vi "LSCI332 SetPID.vi"(0 "VISA Rsrc":refnum<visa-resource-name>="GPIB0::12::INSTR", 5 "Boucle(1)":u32(ring) caption="Boucle" items=["Boucle 1", "Boucle 2"], 9 "Paramètres PID":cluster{"P":dbl, "I":dbl, "D":u32}={"P"=1000.0, "I"=0.0, "D"=0} {"D" max=200 step=1; "I" min=0.1 max=1000.0 step=0.1 format="%#.1f"; "P" min=0.1 max=1000.0 step=0.1 format="%#.1f"}, 11 "error in (no error)":errorcluster) -> (15 "error out":errorcluster)   [LabVIEW 2019]
doc: "Ce VI écrit les paramètres de la zone de contrôle spécifiée dans le contrôlleur"
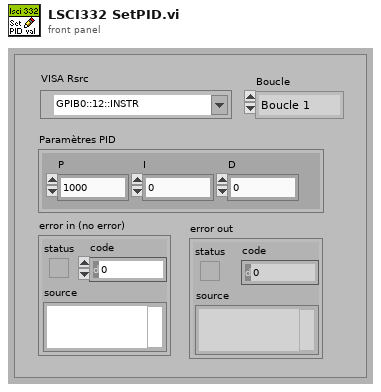
[diagram p1: front panel]
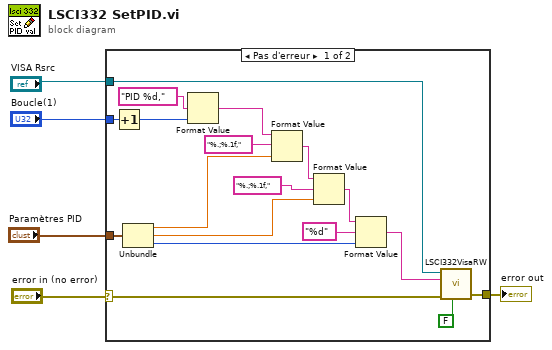
[diagram p0: block diagram]
diagram:
  n1 = case shown="Pas d'erreur" "error in (no error)" {
    selector: "error in (no error)" -> [w11 w24]
    tunnel: "VISA Rsrc" -> [w23 _]
    tunnel: "Boucle(1)" -> [w21 _]
    tunnel: [w22 w24] -> w3
    tunnel: "Paramètres PID" -> [w15 _]
    frame No Error {
      n2 = Increment(x=w21) -> (x+1=w16:u32)
      n3 = Unbundle(w15) -> ("P"=w14:dbl, "I"=w13:dbl, "D"=w12:u32)
      n4 = Format Value(format string="PID %d,", value (0)=w16) -> (output string=w9:string)  [unwired: 1 in]
      n5 = Format Value(string ("")=w9, format string="%.;%.1f,", value (0)=w14) -> (output string=w18:string)
      n6 = Format Value(string ("")=w18, format string="%.;%.1f,", value (0)=w13) -> (output string=w17:string)
      n7 = Format Value(string ("")=w17, format string="%d", value (0)=w12) -> (output string=w8:string)
      n8 = call <userlib>:"LSCI332VisaRW.vi"("Lecture?(T)"=FALSE, "error in (no error)"=w11, "ChaineCom"=w8, "VISA Rsrc"=w23) -> ("error out"=w22:errorcluster)  [unwired: 3 in, 3 out]
    }
    frame Error {
    }
  }
  "error out" <- w3
